vi "MainUI 17.vi"() -> ()   [LabVIEW 2013]
uses:
  eng/trunk/ni/cRIO Master Files/Controls/StateMachineTypeDef.ctl
  eng/trunk/ni/cRIO Master Files/Controls/Up.ctl
  eng/trunk/ni/cRIO Master Files/Controls/Down.ctl
  eng/trunk/ni/cRIO Master Files/Controls/LogState.ctl
  <userlib>/ELL/EventLog/EventLog.lvclass
  <vilib>/Analysis/NI_AALBase.lvlib
  <vilib>/Analysis/3filter.llb/Filter Passband Type.ctl
  <userlib>/ELL/EventLog/Initialize_CSV.vi
  <vilib>/Analysis/3filter.llb/Butterworth Filter (DBL).vi
  eng/trunk/ni/cRIO Master Files/Controls/UserInterfacePages.ctl
  eng/trunk/ni/cRIO Master Files/Controls/SystemControl.ctl
  eng/trunk/ni/cRIO Master Files/Controls/EnergyStorageSelector.ctl
  eng/trunk/ni/cRIO Master Files/Controls/PowerConversionData.ctl
  eng/trunk/ni/cRIO Master Files/Controls/EnergyStorageStringDataArray.ctl
  eng/trunk/ni/cRIO Master Files/Controls/EnergyStorageStringData.ctl
  eng/trunk/ni/cRIO Master Files/Controls/EnergyStorageSystemData.ctl
  eng/trunk/ni/cRIO Master Files/Controls/GensetData.ctl
  Controls/FPGAData.ctl
  eng/trunk/ni/cRIO Master Files/Controls/ModbusInputRegisters.ctl
  eng/trunk/ni/cRIO Master Files/Controls/ModbusHoldingRegisters.ctl
  eng/trunk/ni/cRIO Master Files/Controls/NamedError.ctl
  eng/trunk/ni/cRIO Master Files/Controls/Dial17.ctl
panel:
  in  "Min Cell V":dbl=350.0 min=0.0 max=550.0 format="%#_g V"
  in  "Max Cell V":dbl=672.0 min=3.0 max=750.0 format="%#_g V"
  in  "PS gain P":dbl=0.03
  in  "VI gain P":dbl=55.0
  in  "PS gain I":dbl=0.01
  in  "Cell Limit High":dbl=650.0 min=3.0 max=750.0 format="%#_g V"
  in  "Cell Limit Low":dbl=400.0 min=0.0 max=550.0 format="%#_g V"
  in  "CC gain P":dbl=3.0
  in  "CC gain I":dbl
  in  "HV Setpt":dbl=700.0 format="%#_g V"
  in  "VI gain I":dbl
  in  "Charge Control 2":dbl min=0.0 max=750.0 format="%#_g V"
  in  "Peak Shave 2":dbl min=0.0 max=100.0 format="%#_g kW"
  in  "Up ten PS":T1
  in  "Down ten PS":T2
  in  "Down one PS":T2
  in  "Up one PS":T1
  in  "Up ten MC":T1
  in  "Down ten MC":T2
  in  "Up one MC":T1
  in  "Down one MC":T2
  in  "Manual Current 2":dbl min=-180.0 max=180.0 format="%#_g A"
  in  "Up ten CC":T1
  in  "Down ten CC":T2
  in  "Down one CC":T2
  in  "Up one CC":T1
  out "Samsung":T3
  out "Comap":T3
  out "Interface Data":T3
  out "Log Rate Data":T3
  out "Network Stream":T3
  out "Consumer":T3
  out "Producer":T3
  out "Flush Events":T3
  out "Queue Data Log":T3
  out "Data Logger":T3
  out "DC Voltage":sgl format="%4.1f V"
  out "Samsung Alarm":T4
  out "ComAp Alarm":T4
  out "Siemens Alarm":T4
  in  "Charge Control":bool
  in  "Peak Shave":bool
  out "Exit Program":bool
  in  "Virtual Inertia":bool
  in  "Manual Current":bool
  in  "Stop System":bool
  in  "Start System":bool
  out "Log State":T5
  out "gen eng":u16
  out "gen breaker":u16
  in  "Alarms":bool
  out "Connection Status":bool
  out "Main":bool=TRUE
  in  "Exit Button":bool
  out "Set Points":bool
  out "Metering":bool
  out "Energy Storage":bool
  out "Histogram":bool
  in  "Tab Control":T6=enum."Main"
  out "AC Current 2":sgl(knob) scale=-200.0..200.0 scale format="%3.0fA"
  out "DC Voltage 2":sgl(knob) scale=0.0..750.0 scale format="%3.0fV"
  out "Frequency 2":sgl(knob) scale=45.0..75.0 scale format="%3.0fHz"
  out "DC Current 2":sgl(knob) scale=-200.0..200.0 scale format="%3.0fA"
  out "DC Voltage 3":sgl(knob)=126.0 scale=0.0..750.0 scale format="%3.0fV"
  out "State of Charge":T7=18.015554 scale=0.0..100.0 scale format="%3.0f%"
  out "AC Current":sgl(graph)
  out "Generator Power":sgl(graph)
  out "Generator Frequency":sgl(graph)
  out "Modbus Input Registers":T8 {"Generator Fault Code (30204)" format="%016b"; "Generator Alarm Code (30104)" format="%016b"; "Solar Inverter Fault Code (30203)" format="%016b"; "System Control Fault Code (30202)" format="%016b"; "Power Converter Fault Code (30201)" format="%0d"; "Energy Storage Fault Code (30200)" format="%016b"; "Solar Inverter Alarm Code (30103)" format="%016b"; "System Control Alarm Code (30102)" format="%016b"; "Power Converter Alarm Code (30101)" format="%0d"; "Energy Storage Alarm Code (30100)" format="%016b"; "Fault Word (30053)" format="%016b"; "Alarm Word (30052)" format="%016b"; "Status Word (30051)" format="%016b"}
  out "Modbus Holding Registers":T9={"System Available Capacity (40000)"=600, "System Reserve Percentage (40001)"=200, "System Active Load (40002)"=0, "System Reactive Load (40003)"=0, "Manual Power (40004)"=0, "Manual Current (40005)"=0, "System Watchdog (40006)"=0, "Control Word (40051)"=128, "Clear Faults (40052)"=0} {"Clear Faults (40052)" format="%016b"; "Control Word (40051)" format="%016b"}
  out "Real Time State":string
  out "Drive State":string
  out "E-Stop 2":i32
  out "switch_vert":bool
  out "Power":sgl format="%6.1f kW"
  out "AC Voltage":sgl format="%4.1f V"
  out "icon_batt":bool
  out "switch_batt":bool
  out "switch_gen":bool
  out "switch_drive":bool
  out "switch_load":bool
  out "icon_genset":bool
  out "icon_drive":bool
  out "icon_load":bool
  out "Charge":sgl format="%6.1f %"
  out "DC Current":sgl format="%4.1f A"
  out "DC Voltage":sgl format="%4.1f V"
  out "DC Voltage":sgl format="%4.1f V"
  out "AC Current":sgl format="%4.1f A"
  out "Battery":sgl format="%4.1f V"
  out "Power":dbl format="%6.1f kW"
  out "Frequency":sgl format="%6.1f Hz"
  out "Load":sgl format="%6.1f %"
  out "Temperature":sgl format="%6.1f C"
  out "Power":dbl format="%6.1f kW"
  in  "Clear Alarms":bool
  in  "Stop Log":bool
  out "Alarm Display":string[](array[string])
  out "Alarm Loop":bool
  out "E-Stop":bool
  out "ES System Data":T10
  out "ES String Data":T11
  out "PC Data":T13
  out "FPGA Data":T14
  # "Control Panel"
  # "10"
  # "1"
  # "10"
  # "1"
  # "10"
  # "1"
  # "Charge Limits"
  # "PID Controls"
  # "Energy Storage"
  # "Power Conversion"
  # "System BMS Status"
  # "Rack 1 Status"
  # "Rack 2 Status"
  # "Ioxus UltraCapacitors"
  # "Generator"
  # "Site Load"
  # "Energy Storage"
  # "Power Conversion"
  # "Toshiba"
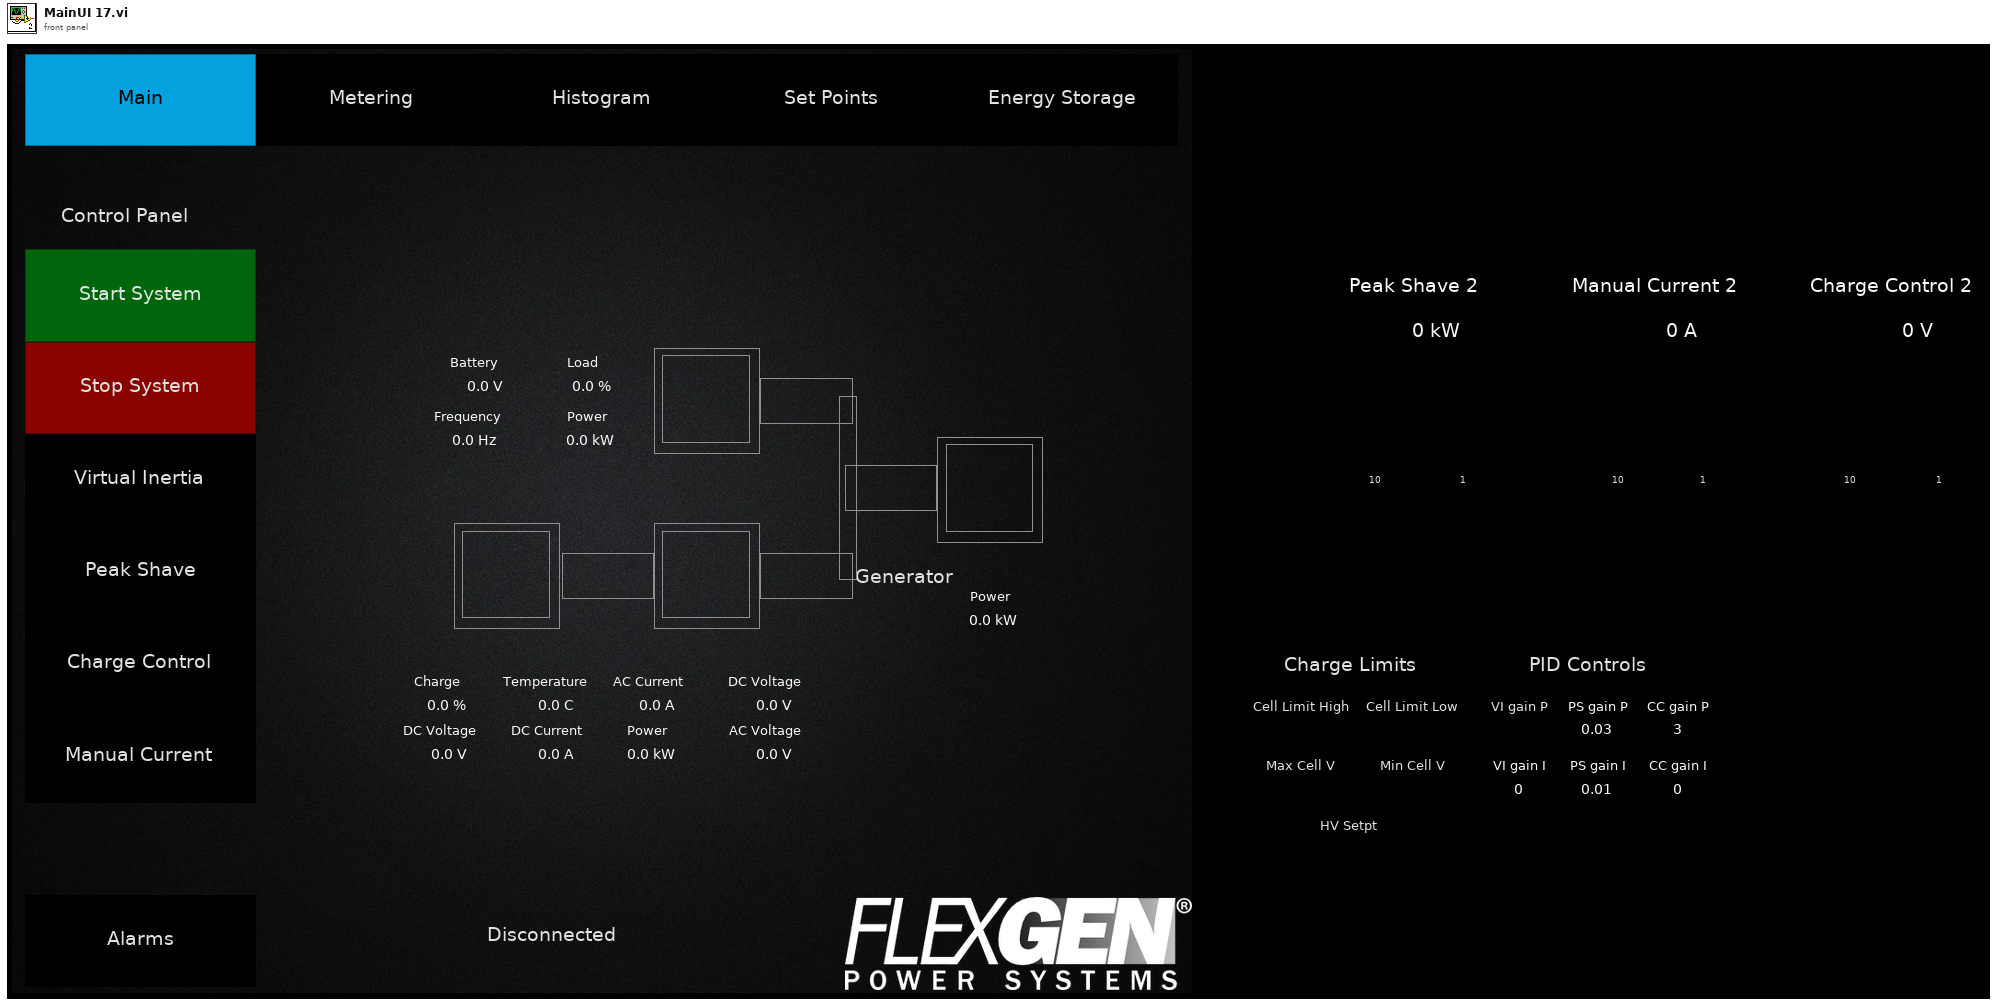
[diagram p1: front panel]
types:
  T1 = typedef "Up.ctl" = bool
  T2 = typedef "Down.ctl" = bool
  T3 = typedef "NamedError.ctl" = cluster{"status":bool, "code":i32, "source":string, "Name":string}
  T4 = cluster{"Fault?":bool, "Alarm?":bool, "Message":string}
  T5 = typedef "LogState.ctl" = enum16{"Rotate Log", "Log Data", "Wait", "Close File", "Generate Filename", "Create New File"}
  T6 = typedef "UserInterfacePages.ctl" = enum32{"Metering", "Histogram", "Set Points", "Samsung", "Ioxus", "Main", "Alarms", "Toshiba", "Siemens"}
  T7 = typedef "Dial17.ctl" = sgl
  T8 = typedef "ModbusInputRegisters.ctl" = cluster{"Energy Remaining (30000)":u16, "Charging Time Remaining (30001)":u16, "Discharging Time Remaining (30002)":u16, "Energy Storage Voltage (30003)":u16, "Energy Storage Current (30004)":i16, "SSG Frequency (30005)":u16, "SSG Total Voltage (30006)":u16, "SSG Total Active Power (30007)":i16, "SSG Total Apparent Power (30008)":i16, "SSG Active Power (L1) (30009)":i16, "SSG Active Power (L2) (30010)":i16, "SSG Active Power (L3) (30011)":i16, "SSG Apparent Power (L1) (30012)":i16, "SSG Apparent Power (L2) (30013)":i16, "SSG Apparent Power (L3) (30014)":i16, "SSG Output Voltage (L1-L2) (30015)":u16, "SSG Output Voltage (L2-L3) (30016)":u16, "SSG Output Voltage (L3-L1) (30017)":u16, "SSG Output Voltage (L1) (30018)":u16, "SSG Output Voltage (L2) (30019)":u16, "SSG Output Voltage (L3) (30020)":u16, "SSG Output Current (L1) (30021)":i16, "SSG Output Current  (L2) (30022)":i16, "SSG Output Current (L3) (30023)":i16, "Energy Storage Temperature (30024)":i16, "Power Converter Temperature (30025)":i16, "Solar Inverter Power (30026)":u16, "Gen Frequency (30027)":u16, "Gen Total Voltage (30028)":u16, "Gen Total Active Power (30029)":i16, "Gen Total Apparent Power (30030)":i16, "Gen Active Power (L1) (30031)":i16, "Gen Active Power (L2) (30032)":i16, "Gen Active Power (L3) (30033)":i16, "Gen Apparent Power (L1) (30034)":i16, "Gen Apparent Power (L2) (30035)":i16, "Gen Apparent Power (L3) (30036)":i16, "Gen Output Voltage (L1-L2) (30037)":u16, "Gen Output Voltage (L2-L3) (30038)":u16, "Gen Output Voltage (L3-L1) (30039)":u16, "Gen Output Voltage (L1) (30040)":u16, "Gen Output Voltage (L2) (30041)":u16, "Gen Output Voltage (L3) (30042)":u16, "Gen Output Current (L1) (30043)":i16, "Gen Output Current  (L2) (30044)":i16, "Gen Output Current (L3) (30045)":i16, "Software Revision (30050)":u16, "Status Word (30051)":u16, "Alarm Word (30052)":u16, "Fault Word (30053)":u16, "Energy Storage Alarm Code (30100)":u16, "Power Converter Alarm Code (30101)":u16, "System Control Alarm Code (30102)":u16, "Solar Inverter Alarm Code (30103)":u16, "Energy Storage Fault Code (30200)":u16, "Power Converter Fault Code (30201)":u16, "System Control Fault Code (30202)":u16, "Solar Inverter Fault Code (30203)":u16, "Generator Alarm Code (30104)":u16, "Generator Fault Code (30204)":u16}
  T9 = typedef "ModbusHoldingRegisters.ctl" = cluster{"System Available Capacity (40000)":u16, "System Reserve Percentage (40001)":u16, "System Active Load (40002)":i16, "System Reactive Load (40003)":i16, "Manual Power (40004)":i16, "Manual Current (40005)":i16, "System Watchdog (40006)":u16, "Control Word (40051)":u16, "Clear Faults (40052)":u16}
  T10 = typedef "EnergyStorageSystemData.ctl" = cluster{"Voltage":sgl, "Current":sgl, "SOC Avg":sgl, "Faults":u16, "Alarms":u16, "Number of Strings":u16, "Max Temp":i16, "Min Temp":i16, "Max Cell Voltage":sgl, "Min Cell Voltage":sgl, "Energy Capacity (kWh)":sgl, "Energy Remaining (kWh)":sgl, "String Code":u16, "SOC Min":sgl, "SOC Max":sgl}
  T11 = typedef "EnergyStorageStringDataArray.ctl" = T12[]
  T12 = typedef "EnergyStorageStringData.ctl" = cluster{"Voltage":sgl, "State of Charge":sgl, "Current":sgl, "Temperature Min":i16, "Temperature Max":i16, "Faults":u16, "Alarms":u16, "String Number":u16, "Contactor Status":bool, "String Ready?":bool, "Cells Balancing":bool, "Cell V Max":dbl, "Cell V Min":dbl}
  T13 = typedef "PowerConversionData.ctl" = cluster{"Active Power":sgl, "Reactive Power":sgl, "AC Current":sgl, "DC Current":sgl, "AC Voltage":sgl, "DC Voltage":sgl, "Temperature":sgl, "Alarms":u16, "Faults":u16, "Status":u16}
  T14 = typedef "FPGAData.ctl" = cluster{"SSG Frequency":sgl, "SSG Total Voltage":dbl, "SSG Active Power":sgl, "SSG Apparent Power":sgl, "SSG Active Power (L1)":dbl, "SSG Active Power (L2)":dbl, "SSG Active Power (L3)":dbl, "SSG Apparent Power (L1)":dbl, "SSG Apparent Power (L2)":dbl, "SSG Apparent Power (L3)":dbl, "SSG Vrms (L1-L2)":dbl, "SSG Vrms (L2-L3)":dbl, "SSG Vrms (L3-L1)":dbl, "SSG Vrms (L1)":dbl, "SSG Vrms (L2)":dbl, "SSG Vrms (L3)":dbl, "SSG Arms (L1)":dbl, "SSG Arms (L2)":dbl, "SSG Arms (L3)":dbl, "Gen Frequency":sgl, "Gen Total Voltage":dbl, "Gen Active Power":sgl, "Gen Apparent Power":sgl, "Gen Active Power (L1)":dbl, "Gen Active Power (L2)":dbl, "Gen Active Power (L3)":dbl, "Gen Apparent Power (L1)":dbl, "Gen Apparent Power (L2)":dbl, "Gen Apparent Power (L3)":dbl, "Gen Vrms (L1-L2)":dbl, "Gen Vrms (L2-L3)":dbl, "Gen Vrms (L3-L1)":dbl, "Gen Vrms (L1)":dbl, "Gen Vrms (L2)":dbl, "Gen Vrms (L3)":dbl, "Gen Arms (L1)":dbl, "Gen Arms (L2)":dbl, "Gen Arms (L3)":dbl, "ES Vdc 1":sgl, "ES Vdc 2":sgl, "Load %":sgl, "Load Imbalance %":sgl, "E-Stop":bool, "Battle Short":bool, "Auto Start":bool, "Gen Contactor":bool, "ES Relay 1":bool, "ES Relay 2":bool, "NFT-N Contactor":bool, "NFT-G Contactor ":bool, "ES Relay 3":bool, "ES Relay 4":bool, "ES Relay 5":bool, "ES Relay 6":bool, "ES Vdc 3":sgl, "ES Vdc 4":sgl, "ES Vdc 5":sgl, "ES Vdc 6":sgl}
  T15 = typedef "StateMachineTypeDef.ctl" = enum16{"Idle", "Initialize", "Alarm Clicked", "go to Set Points", "go to Energy Storage", "go to Power Conversion ", "go to Histogram", "go to Main", "go to Metering", "Enable Charge Control", "Enable External Control", "Enable Manual Current", "Enable Peak Shave", "Disable Virtual Inertia", "Start System", "Stop System", "Shutdown", "Error"}
  T16 = typedef "EnergyStorageSelector.ctl" = enum16{"Other", "Toshiba", "Ioxus", "Samsung"}
  T17 = typedef "NI_AALBase.lvlib/Filter Passband Type.ctl" = enum32{"Lowpass", "Highpass", "Bandpass", "Bandstop"}
  T18 = typedef "FPGAData.ctl" = cluster{"SSG Frequency":sgl, "SSG Total Voltage":dbl, "SSG Active Power":sgl, "SSG Apparent Power":sgl, "SSG Active Power (L1)":dbl, "SSG Active Power (L2)":dbl, "SSG Active Power (L3)":dbl, "SSG Apparent Power (L1)":dbl, "SSG Apparent Power (L2)":dbl, "SSG Apparent Power (L3)":dbl, "SSG Vrms (L1-L2)":dbl, "SSG Vrms (L2-L3)":dbl, "SSG Vrms (L3-L1)":dbl, "SSG Vrms (L1)":dbl, "SSG Vrms (L2)":dbl, "SSG Vrms (L3)":dbl, "SSG Arms (L1)":dbl, "SSG Arms (L2)":dbl, "SSG Arms (L3)":dbl, "Gen Frequency":sgl, "Gen Total Voltage":dbl, "Gen Active Power":sgl, "Gen Apparent Power":sgl, "Gen Active Power (L1)":dbl, "Gen Active Power (L2)":dbl, "Gen Active Power (L3)":dbl, "Gen Apparent Power (L1)":dbl, "Gen Apparent Power (L2)":dbl, "Gen Apparent Power (L3)":dbl, "Gen Vrms (L1-L2)":dbl, "Gen Vrms (L2-L3)":dbl, "Gen Vrms (L3-L1)":dbl, "Gen Vrms (L1)":dbl, "Gen Vrms (L2)":dbl, "Gen Vrms (L3)":dbl, "Gen Arms (L1)":dbl, "Gen Arms (L2)":dbl, "Gen Arms (L3)":dbl, "ES Vdc String 1":sgl, "ES Vdc String 2":sgl, "Load %":sgl, "Load Imbalance %":sgl, "E-Stop":bool, "Battle Short":bool, "Auto Start":bool, "Gen Contactor":bool, "Battery Relay 1":bool, "Battery Relay 2":bool, "NFT-N Contactor":bool, "NFT-G Contactor ":bool}
  T19 = typedef "GensetData.ctl" = cluster{"Alarm Array":u16[], "Power":i16, "Frequency":u16, "Battery":i16, "Engine State":u16, "Breaker State":u16, "Load %":i16}
  T20 = cluster{"status":bool, "code":i32, "source":string, "Name":string}[]
  T21 = cluster{"Fault?":bool, "Alarm?":bool, "Message":string}[]
  T22 = typedef "SystemControl.ctl" = cluster{"Start":bool, "Stop":bool, "Power System Enable":bool, "SSG Control":bool, "Virtual Inertia":bool, "Manual Current":bool, "Peak Shave":bool, "Spot Generation":bool, "Charge Control":bool, "Watchdog":bool, "ComAp Fault":bool, "Clear Gen Faults":bool, "Clear PV Faults":bool, "Clear System Faults":bool, "Clear PC Faults":bool, "Clear ES Faults":bool, "Clear Watchdog Faults":bool, "Peak Shave Value":dbl, "Manual Current Value":dbl, "Charge Control Value":dbl, "Gen Capacity":dbl, "Gen Reserve":dbl, "VI gain P":dbl, "CC gain P":dbl, "CC gain I":dbl}
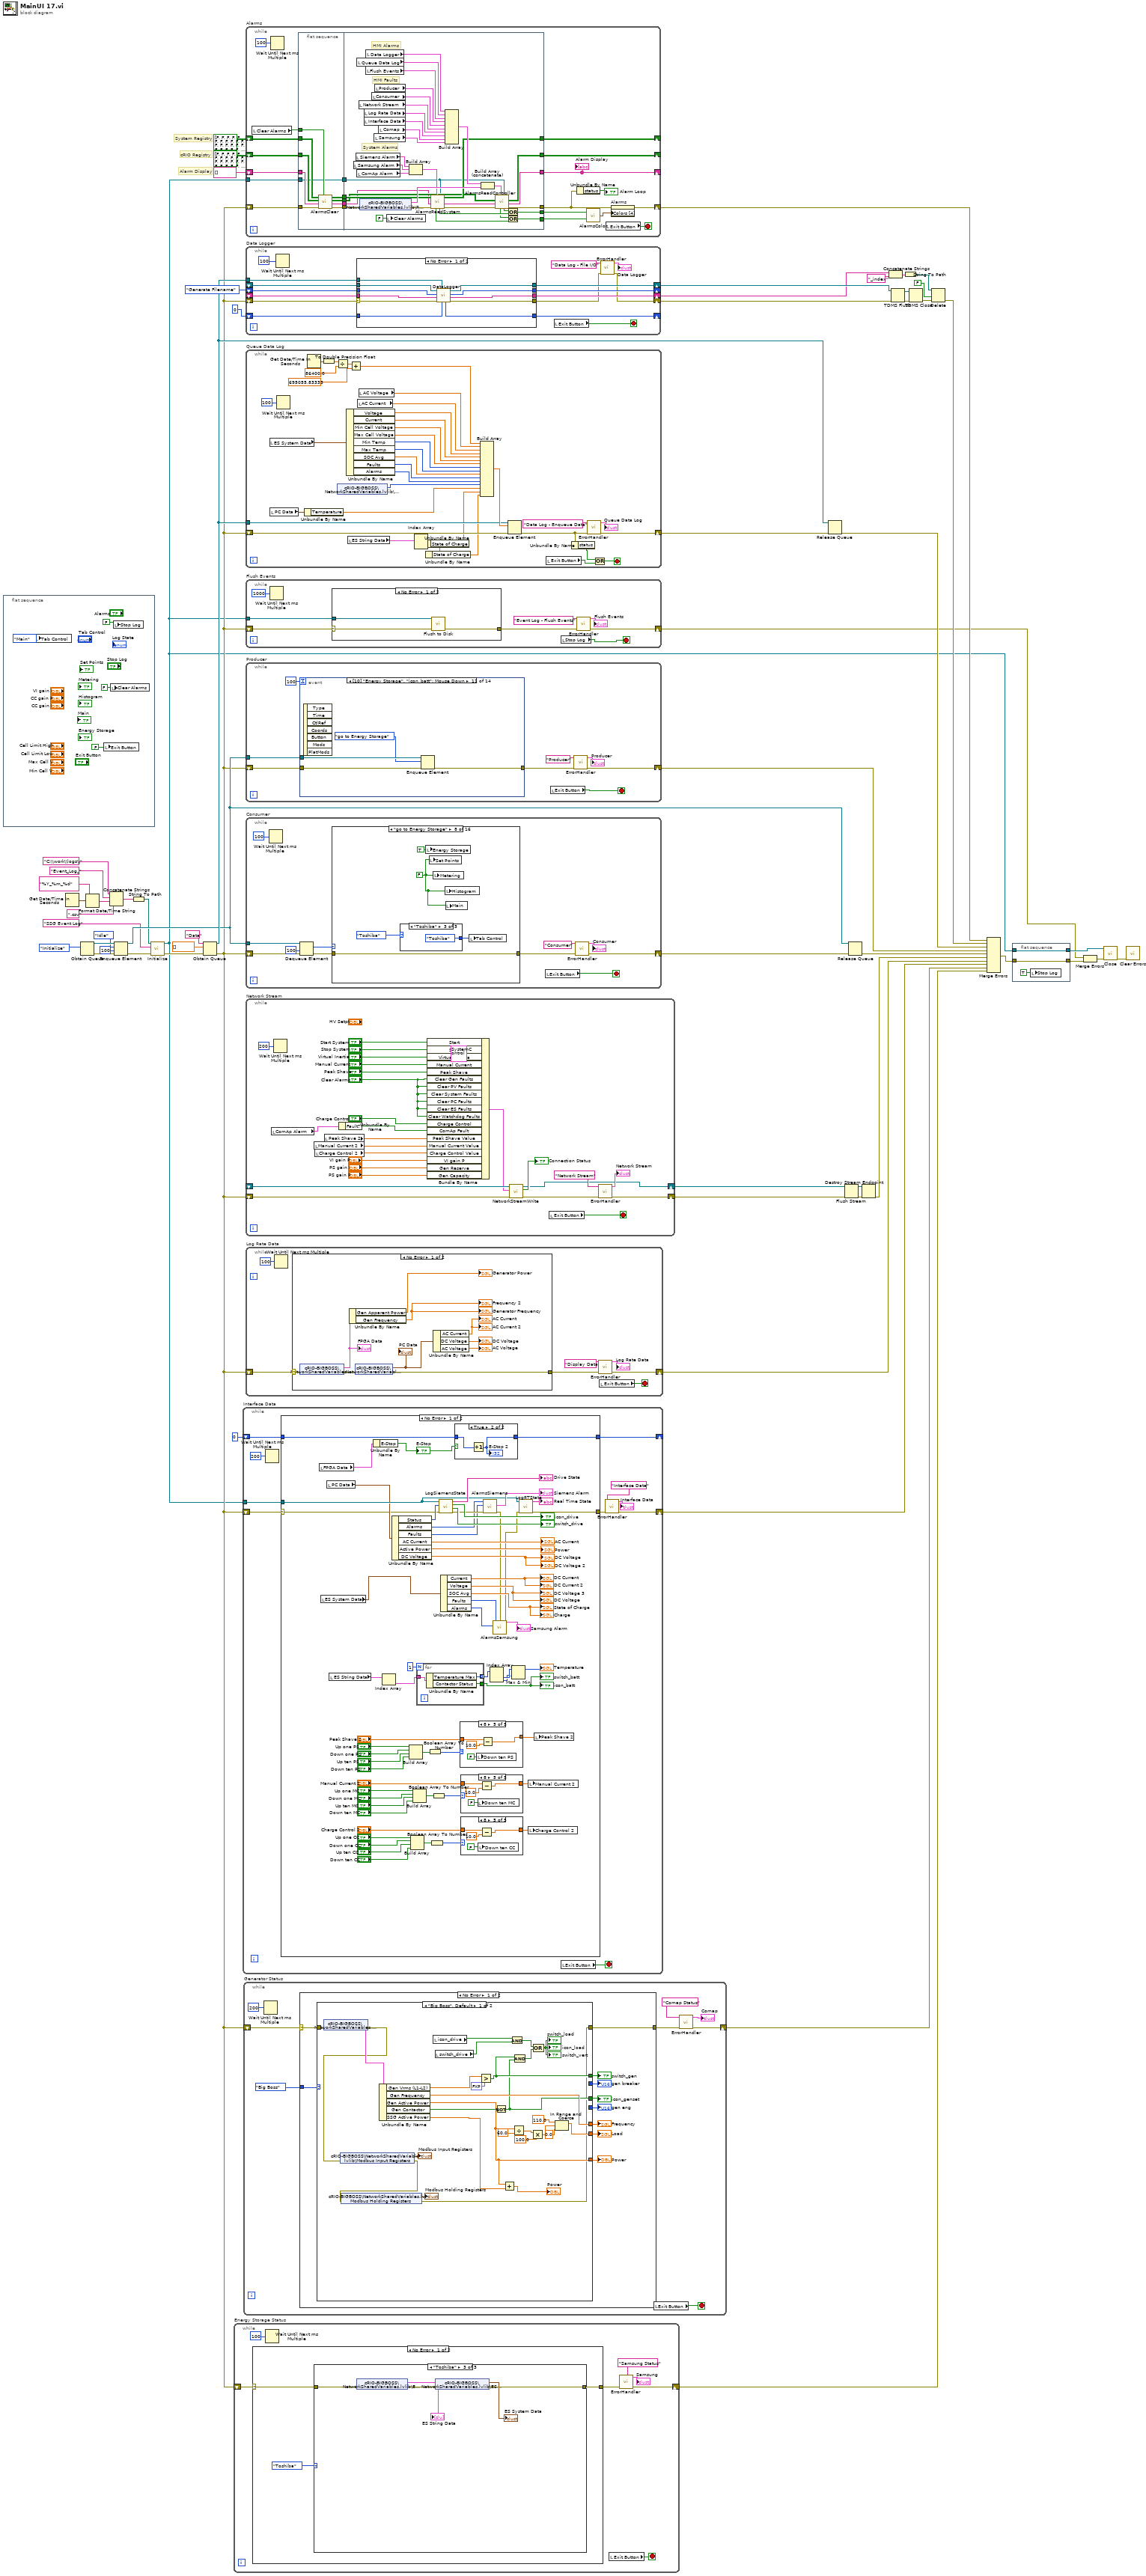
[diagram p0: block diagram]
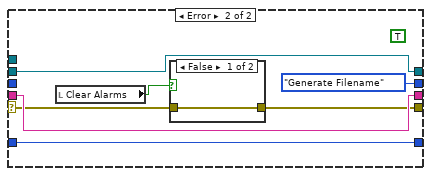
[diagram p2: hidden frame]
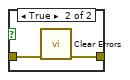
[diagram p3: hidden frame]
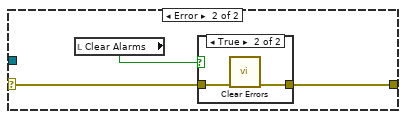
[diagram p4: hidden frame]
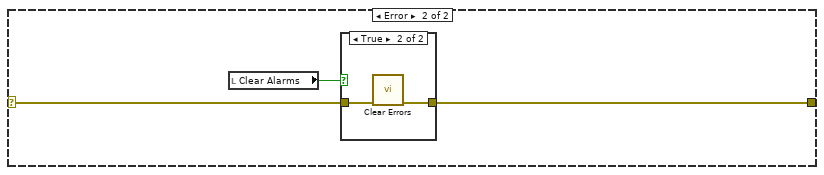
[diagram p8: hidden frame]
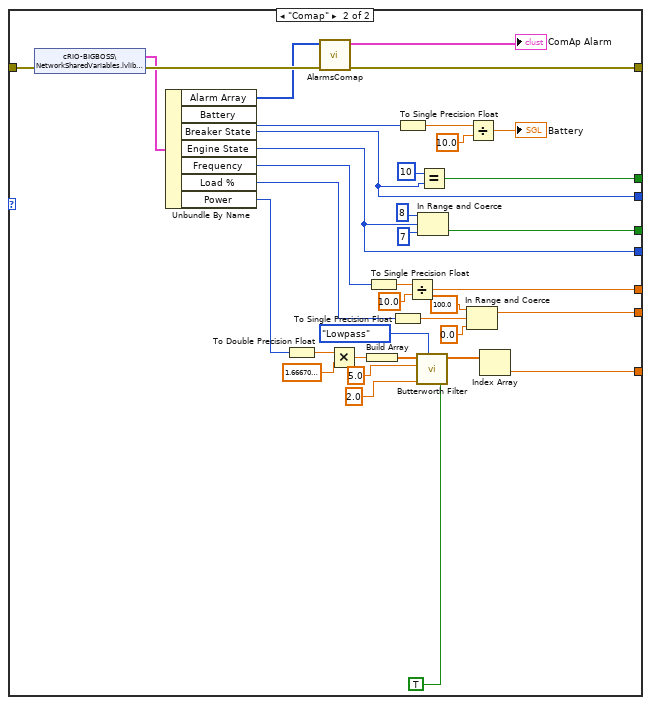
[diagram p10: hidden frame]
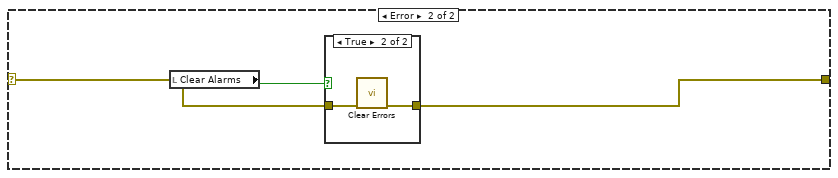
[diagram p11: hidden frame]
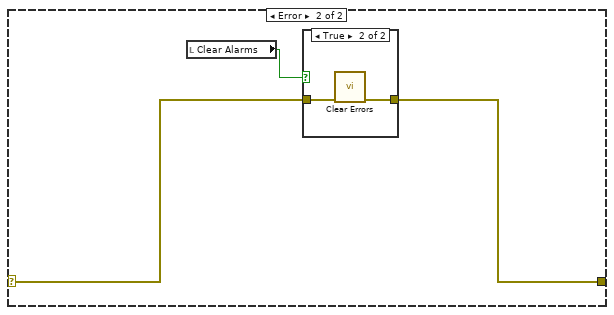
[diagram p13: hidden frame]
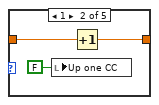
[diagram p16: hidden frame]
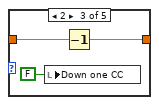
[diagram p17: hidden frame]
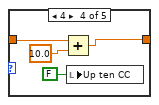
[diagram p18: hidden frame]
diagram:
  # "Alarm Display"
  # "System Registry"
  # "cRIO Registry"
  n1 = flat-sequence {
    frame #0 {
      n2 = local write "Tab Control"(UserInterfacePages."Main" ("Tab Control")) -> ()
      n3 = local write "Exit Button"(FALSE ("Stop Button")) -> ()
      n4 = local write "Clear Alarms"(FALSE ("Clear Errors")) -> ()
      n5 = local write "Stop Log"(FALSE ("Stop Log")) -> ()
    }
  }
  n6 = Get Date/Time In Seconds() -> (seconds since 1Jan1904=w38:timestamp)
  n7 = Obtain Queue(element data type=StateMachineTypeDef."Initialize") -> (queue out=w58:refnum<queue>, error out=w59:errorcluster)  [unwired: 4 in, 1 out]
  n8 = Format Date/Time String(time format string (%c)="%Y_%m_%d", seconds (now)=w38) -> (date/time string=w37:string)  [unwired: 1 in]
  n9 = Concatenate Strings("C:\\work\\logs\\" ("string"), "Event_Log_" ("string"), w37, ".csv" ("string")) -> (w35:string)
  n10 = Enqueue Element(queue=w58, element=StateMachineTypeDef."Idle", timeout in ms (-1)=100, error in (no error)=w59) -> (queue out=w36:refnum<queue>, error out=w27:errorcluster)  [unwired: 1 out]
  n11 = String To Path(string=w35) -> (path=w34:path)
  n12 = call-poly <userlib>:"Initialize.vi"("error in (no error)"=w27, "Description"="SSG Event Log", "Path"=w34) -> ("error out"=w26:errorcluster, "EventLog ref"=w1:refnum<class "EventLog.lvclass">)  [unwired: 7 in]
  n13 = Obtain Queue(name (unnamed)="Data", element data type=dbl[] [] ("appended array"), error in (no error)=w26) -> (queue out=w48:refnum<queue>, error out=w13:errorcluster)  [unwired: 2 in, 1 out]
  n14 = while "Energy Storage Status" {
    shift-right: [w65] -> w19
    shift-left: w13 -> [w69]
    stop <- w70 stop-if-true
    n15 = case shown="No Error" w69 {
      selector: w69 -> [w73 w83]
      tunnel: [w74 w82] -> w68
      frame No Error {
        n16 = case shown="\"Toshiba\"" EnergyStorageSelector."Toshiba" ("Energy Storage Selector") {
          tunnel: w73 -> [w75 w76 w79]
          tunnel: [w75 w76 w81] -> w74
          frame "Other", Default {
          }
          frame "Samsung" {
          }
          frame "Toshiba" {
            n17 = shared-variable "cRIO-BIGBOSS\\NetworkSharedVariables.lvlib\\ES String Data"(error in=w79) -> (→"ES String Data":T11, error out=w78:errorcluster)
            n18 = shared-variable "cRIO-BIGBOSS\\NetworkSharedVariables.lvlib\\ES System Data"(error in=w78) -> (→"ES System Data":T10, error out=w81:errorcluster)
          }
        }
      }
      frame Error {
        n19 = local read "Clear Alarms"() -> (w84:bool)
        n20 = case shown="True" w84 {
          tunnel: w83 -> [w85 w87]
          tunnel: [w85 w86] -> w82
          frame False {
          }
          frame True {
            n21 = call <vilib>:"Clear Errors.vi"("error in (no error)"=w87) -> ("error out"=w86:errorcluster)  [unwired: 6 in]
          }
        }
      }
    }
    n22 = Wait Until Next ms Multiple(millisecond multiple=u32 100 ("milliseconds to wait")) -> ()  [unwired: 1 out]
    n23 = local read "Exit Button"() -> (w70:bool)
    n24 = call "ErrorHandler.vi"("Error In"=w68, "Name"="Samsung Status") -> ("Error Out"=w65:errorcluster, "Named Error Out"=→"Samsung":T3)  [unwired: 6 in]
  }
  n25 = while "Interface Data" {
    shift-right: [w88] -> w14
    shift-left: w13 -> [w94]
    tunnel: w1 -> [w96]
    shift-right: [w92] -> _
    shift-left: 0 -> [w93]
    stop <- w95 stop-if-true
    n26 = Wait Until Next ms Multiple(millisecond multiple=u32 200 ("milliseconds to wait")) -> ()  [unwired: 1 out]
    n27 = case shown="No Error" w94 {
      selector: w94 -> [w98 w211]
      tunnel: w96 -> [w126 _]
      tunnel: [w132 w210] -> w90
      tunnel: w93 -> [w142 w213]
      tunnel: [w141 w213] -> w92
      frame No Error {
        n28 = local read "FPGA Data"() -> (w99:T14)
        n29 = local read "ES System Data"() -> (w104:T10)
        n30 = local read "PC Data"() -> (w100:T13)
        n31 = local read "ES String Data"() -> (w103:T11)
        n32 = Unbundle By Name(w99) -> ("E-Stop"=w105:bool)
        "E-Stop" <- w105
        n33 = Index Array(array=w103) -> (element=w102:T12)  [unwired: 1 in]
        n34 = Unbundle By Name(w100) -> ("Status"=w111:u16, "Alarms"=w112:u16, "Faults"=w113:u16, "AC Current"=→"AC Current":sgl, "Active Power"=→"Power":sgl, "DC Voltage"=→"DC Voltage" →"DC Voltage 2":sgl)
        n35 = Build Array("Up one PS", "Down one PS", "Up ten PS", "Down ten PS") -> (w146:T2[])
        n36 = Build Array("Up one CC", "Down one CC", "Up ten CC", "Down ten CC") -> (w136:T2[])
        n37 = Build Array("Up one MC", "Down one MC", "Up ten MC", "Down ten MC") -> (w153:T2[])
        n38 = for {
          N: 1 -> [_]
          tunnel: w102 -> [w161]
          tunnel: [w160] -> w117 mode=indexing
          tunnel: [w159] -> w114
          n39 = Unbundle By Name(w161) -> ("Temperature Max"=w160:i16, "Contactor Status"=w159:bool)
        }
        "switch_batt" <- w114
        "icon_batt" <- w114
        n40 = Boolean Array To Number(Boolean array=w146) -> (number=w145:u32)
        n41 = Boolean Array To Number(Boolean array=w136) -> (number=w135:u32)
        n42 = Boolean Array To Number(Boolean array=w153) -> (number=w154:u32)
        n43 = call "LogSiemensState.vi"("Error In"=w98, "pb Status In"=w111, "EventLog ref"=w126) -> ("Error Out"=w125:errorcluster, "Switch Out"=→"switch_drive":bool, "Icon Out"=→"icon_drive":bool, "State Out"=→"Drive State":string)  [unwired: 1 in]
        n44 = Unbundle By Name(w104) -> ("Current"=→"DC Current" →"DC Current 2":sgl, "Voltage"=→"DC Voltage" →"DC Voltage 3":sgl, "SOC Avg"=→"Charge" →"State of Charge":sgl, "Faults"=w109:u16, "Alarms"=w108:u16)
        n45 = case shown="True" w105 {
          tunnel: w142 -> [w177 w179]
          tunnel: [w177 w178] -> w141
          frame False {
          }
          frame True {
            n46 = Increment(x=w179) -> (x+1=w178:i32)
            "E-Stop 2" <- w178
          }
        }
        n47 = case shown="8" w145 {
          tunnel: [w180 w183 w186 w189 w194] -> w144
          tunnel: "Peak Shave 2" -> [w180 w181 w184 w187 w191]
          frame 0, Default {
          }
          frame 1 {
            n48 = Increment(x=w181) -> (x+1=w183:dbl)
            n49 = local write "Up one PS"(T1 FALSE ("Up one 2")) -> ()
          }
          frame 2 {
            n50 = local write "Down one PS"(T2 FALSE ("Down one 2")) -> ()
            n51 = Decrement(x=w184) -> (x-1=w186:dbl)
          }
          frame 4 {
            n52 = Add(x=w187, y=10.0) -> (x+y=w189:dbl)
            n53 = local write "Up ten PS"(T1 FALSE ("Up ten 2")) -> ()
          }
          frame 8 {
            n54 = local write "Down ten PS"(T2 FALSE ("Down ten 2")) -> ()
            n55 = Subtract(x=w191, y=10.0) -> (x-y=w194:dbl)
          }
        }
        n56 = case shown="8" w154 {
          tunnel: [w195 w196 w200 w202 w207] -> w152
          tunnel: "Manual Current 2" -> [w195 w197 w201 w204 w208]
          frame 0, Default {
          }
          frame 1 {
            n57 = local write "Up one MC"(T1 FALSE ("Up one")) -> ()
            n58 = Increment(x=w197) -> (x+1=w196:dbl)
          }
          frame 2 {
            n59 = local write "Down one MC"(T2 FALSE ("Down one")) -> ()
            n60 = Decrement(x=w201) -> (x-1=w200:dbl)
          }
          frame 4 {
            n61 = local write "Up ten MC"(T1 FALSE ("Up ten")) -> ()
            n62 = Add(x=w204, y=10.0) -> (x+y=w202:dbl)
          }
          frame 8 {
            n63 = local write "Down ten MC"(T2 FALSE ("Down ten")) -> ()
            n64 = Subtract(x=w208, y=10.0) -> (x-y=w207:dbl)
          }
        }
        n65 = case shown="8" w135 {
          tunnel: "Charge Control 2" -> [w162 w165 w168 w172 w176]
          tunnel: [w162 w164 w167 w171 w174] -> w133
          frame 0, Default {
          }
          frame 1 {
            n66 = local write "Up one CC"(T1 FALSE ("Up one CC")) -> ()
            n67 = Increment(x=w165) -> (x+1=w164:dbl)
          }
          frame 2 {
            n68 = local write "Down one CC"(T2 FALSE ("Down one CC")) -> ()
            n69 = Decrement(x=w168) -> (x-1=w167:dbl)
          }
          frame 4 {
            n70 = Add(x=w172, y=10.0) -> (x+y=w171:dbl)
            n71 = local write "Up ten CC"(T1 FALSE ("Up ten CC")) -> ()
          }
          frame 8 {
            n72 = local write "Down ten CC"(T2 FALSE ("Down ten CC")) -> ()
            n73 = Subtract(x=w176, y=10.0) -> (x-y=w174:dbl)
          }
        }
        n74 = call "AlarmsSiemens.vi"("Error In"=w125, "pb Fault Code"=w113, "pb Alarm Code"=w112) -> ("Error Out"=w107:errorcluster, "System Alarm Out"=→"Siemens Alarm":T4)  [unwired: 3 in]
        n75 = Index Array(array=w117) -> (element #1=w116:i16, element #2=w115:i16)  [unwired: 2 in]
        n76 = call "AlarmsSamsung.vi"("Error In"=w107, "Alarm Code"=w108, "Fault Code"=w109) -> ("Error Out"=w106:errorcluster, "System Alarm Out"=→"Samsung Alarm":T4)  [unwired: 5 in]
        n77 = Max & Min(x=w116, y=w115) -> (max(x,y)=→"Temperature":i16)  [unwired: 1 out]
        n78 = call "LogRTState.vi"("Error In"=w106, "EventLog ref"=w126) -> ("Error Out"=w132:errorcluster, "State Out"=→"Real Time State":string)  [unwired: 4 in]
        n79 = local write "Manual Current 2"(w152) -> ()
        n80 = local write "Charge Control 2"(w133) -> ()
        n81 = local write "Peak Shave 2"(w144) -> ()
      }
      frame Error {
        n82 = local read "Clear Alarms"() -> (w212:bool)
        n83 = case shown="False" w212 {
          tunnel: [w214 w216] -> w210
          tunnel: w211 -> [w214 w215]
          frame False {
          }
          frame True {
            n84 = call <vilib>:"Clear Errors.vi"("error in (no error)"=w215) -> ("error out"=w216:errorcluster)  [unwired: 6 in]
          }
        }
      }
    }
    n85 = local read "Exit Button"() -> (w95:bool)
    n86 = call "ErrorHandler.vi"("Error In"=w90, "Name"="Interface Data") -> ("Error Out"=w88:errorcluster, "Named Error Out"=→"Interface Data":T3)  [unwired: 6 in]
  }
  n87 = while "Generator Status" {
    shift-right: [w218] -> w20
    shift-left: w13 -> [w222]
    stop <- w223 stop-if-true
    n88 = Wait Until Next ms Multiple(millisecond multiple=u32 200 ("milliseconds to wait")) -> ()  [unwired: 1 out]
    n89 = case shown="No Error" w222 {
      selector: w222 -> [w229 w302]
      tunnel: [w226 w301] -> w221
      tunnel: enum16{"Big Boss", "Comap"}."Big Boss" -> [w225 _]
      frame No Error {
        n90 = case shown="\"Big Boss\", Default" w225 {
          tunnel: [w256 w299] -> w234
          tunnel: [w252 w294] -> w233
          tunnel: [w246 w288] -> w232
          tunnel: [w245 w286] -> w231
          tunnel: [w248 w278] -> w230
          tunnel: w229 -> [w262 w273]
          tunnel: [_ w268] -> w228
          tunnel: [_ w267] -> w227
          tunnel: [w237 w263] -> w226
          frame "Big Boss", Default {
            n91 = shared-variable "cRIO-BIGBOSS\\NetworkSharedVariables.lvlib\\FPGA Data"(error in=w262) -> (w261:T18, error out=w239:errorcluster)
            n92 = shared-variable "cRIO-BIGBOSS\\NetworkSharedVariables.lvlib\\Modbus Input Registers"(error in=w239) -> (→"Modbus Input Registers":T8, error out=w238:errorcluster)
            n93 = shared-variable "cRIO-BIGBOSS\\NetworkSharedVariables.lvlib\\Modbus Holding Registers"(error in=w238) -> (→"Modbus Holding Registers":T9, error out=w237:errorcluster)
            n94 = Unbundle By Name(w261) -> ("Gen Vrms (L1-L2)"=w251:dbl, "Gen Frequency"=w252:sgl, "Gen Active Power"=w248:sgl, "Gen Contactor"=w260:bool, "SSG Active Power"=w249:sgl)
            n95 = local read "icon_drive"() -> (w241:bool)
            n96 = local read "switch_drive"() -> (w240:bool)
            n97 = Greater?(x=w251, y=fxp<+,24,10> 160.0) -> (0:w246:bool)
            n98 = Not(x=w260) -> (.not. x?=w245:bool)
            n99 = Add(x=w248, y=w249) -> (x+y=→"Power":sgl)
            n100 = Compound Arithmetic op=AND(w241, w240) -> (w242:bool)
            n101 = Divide(x=w248, y=sgl 60.0) -> (x/y=w258:sgl)
            n102 = Compound Arithmetic op=AND(w246, w245) -> (w244:bool)
            n103 = Multiply(x=w258, y=sgl 100.0) -> (x*y=w255:sgl)
            n104 = Compound Arithmetic op=OR(w242, w244) -> (→"switch_vert" →"switch_load":bool)
            n105 = In Range and Coerce(upper limit=sgl 110.0, x=w255, lower limit=sgl 0.0) -> (coerced(x)=w256:sgl)  [unwired: 1 out]
          }
          frame "Comap" {
            n106 = shared-variable "cRIO-BIGBOSS\\NetworkSharedVariables.lvlib\\Comap Data"(error in=w273) -> (w271:T19, error out=w272:errorcluster)
            n107 = Unbundle By Name(w271) -> ("Alarm Array"=w270:u16[], "Battery"=w269:i16, "Breaker State"=w268:u16, "Engine State"=w267:u16, "Frequency"=w266:u16, "Load %"=w265:i16, "Power"=w264:i16)
            n108 = To Double Precision Float(number=w264) -> (double precision float=w295:dbl)
            n109 = call "AlarmsComap.vi"("Error In"=w272, "Alarm Array"=w270) -> ("Error Out"=w263:errorcluster, "System Alarm Out"=→"ComAp Alarm":T4)  [unwired: 6 in]
            n110 = Multiply(x=w295, y=1.666700005531311) -> (x*y=w281:dbl)
            n111 = Build Array(w281) -> (w280:dbl[])
            n112 = To Single Precision Float(number=w266) -> (single precision float=w292:sgl)
            n113 = To Single Precision Float(number=w265) -> (single precision float=w296:sgl)
            n114 = To Single Precision Float(number=w269) -> (single precision float=w290:sgl)
            n115 = Divide(x=w292, y=sgl 10.0) -> (x/y=w294:sgl)
            n116 = call-poly <vilib>:"Butterworth Filter.vi"("init/cont (init:F)"=TRUE, "filter type"=Filter_Passband_Type."Lowpass", "low cutoff freq: fl"=2.0, "sampling freq: fs"=5.0, "X"=w280) -> ("Filtered X"=w279:dbl[])  [unwired: 3 in, 1 out]
            n117 = In Range and Coerce(upper limit=u16 8, x=w267, lower limit=u16 7) -> (In Range?=w286:bool)  [unwired: 1 out]
            n118 = Equal?(x=u16 10, y=w268) -> (x = y?=w288:bool)
            n119 = In Range and Coerce(upper limit=sgl 100.0, x=w296, lower limit=sgl 0.0) -> (coerced(x)=w299:sgl)  [unwired: 1 out]
            n120 = Divide(x=w290, y=sgl 10.0) -> (x/y=→"Battery":sgl)
            n121 = Index Array(array=w279) -> (element=w278:dbl)  [unwired: 1 in]
          }
        }
        "icon_genset" <- w231
        "switch_gen" <- w232
        "gen breaker" <- w228
        "gen eng" <- w227
        "Power" <- w230
        "Frequency" <- w233
        "Load" <- w234
      }
      frame Error {
        n122 = local read "Clear Alarms"() -> (w300:bool)
        n123 = case shown="True" w300 {
          tunnel: w302 -> [w303 w305]
          tunnel: [w303 w304] -> w301
          frame False {
          }
          frame True {
            n124 = call <vilib>:"Clear Errors.vi"("error in (no error)"=w305) -> ("error out"=w304:errorcluster)  [unwired: 6 in]
          }
        }
      }
    }
    n125 = local read "Exit Button"() -> (w223:bool)
    n126 = call "ErrorHandler.vi"("Error In"=w221, "Name"="Comap Status") -> ("Error Out"=w218:errorcluster, "Named Error Out"=→"Comap":T3)  [unwired: 6 in]
  }
  n127 = while "Alarms" {
    shift-right: [w324] -> w10
    shift-left: w13 -> [w319]
    shift-right: [w314] -> _
    shift-left: string[] [] ("Alarms Display Out") -> [w320]
    shift-right: [w315] -> _
    shift-left: bool[][] [[FALSE, FALSE, FALSE, FALSE, FALSE, FALSE, FALSE, FALSE, FALSE, FALSE, FALSE, FALSE, FALSE, FALSE, FALSE, FALSE, FALSE, FALSE, FALSE, FALSE, FALSE], [FALSE, FALSE, FALSE, FALSE, FALSE, FALSE, FALSE, FALSE, FALSE, FALSE, FALSE, FALSE, FALSE, FALSE, FALSE, FALSE, FALSE, FALSE, FALSE, FALSE, FALSE]] ("Alarm Registry Out") -> [w321]
    shift-right: [w316] -> _
    shift-left: bool[][] [[FALSE, FALSE, FALSE, FALSE, FALSE, FALSE, FALSE, FALSE, FALSE, FALSE, FALSE, FALSE, FALSE, FALSE, FALSE, FALSE, FALSE, FALSE, FALSE, FALSE, FALSE], [FALSE, FALSE, FALSE, FALSE, FALSE, FALSE, FALSE, FALSE, FALSE, FALSE, FALSE, FALSE, FALSE, FALSE, FALSE, FALSE, FALSE, FALSE, FALSE, FALSE, FALSE]] ("Alarm Registry Out") -> [w318]
    tunnel: w1 -> [w306]
    stop <- w327 stop-if-true
    n128 = local read "Clear Alarms"() -> (w322:bool)
    n129 = Wait Until Next ms Multiple(millisecond multiple=u32 100 ("milliseconds to wait")) -> ()  [unwired: 1 out]
    n130 = flat-sequence {
      tunnel: w322 -> [w331]
      tunnel: w321 -> [w333]
      tunnel: w320 -> [w334]
      tunnel: w319 -> [w336]
      tunnel: w318 -> [w332]
      tunnel: [w337] -> w317
      tunnel: [w335] -> w310
      tunnel: [w330] -> w309
      tunnel: [w329] -> w308
      tunnel: w306 -> [w328]
      tunnel: [w328] -> w307
      tunnel: [w344] -> w311
      tunnel: [w350] -> w316
      tunnel: [w345] -> w315
      tunnel: [w339] -> w314
      tunnel: [w372] -> w312
      tunnel: [w373] -> w313
      tunnel: w317 -> [w352]
      tunnel: w310 -> [w371]
      tunnel: w309 -> [w342]
      tunnel: w308 -> [w340]
      tunnel: w307 -> [w338]
      frame #0 {
        n131 = call "AlarmsClear.vi"("Clear Alarms? In"=w331, "Error In"=w336, "Alarm Display In"=w334, "cRIO Registry In"=w333, "System Registry In"=w332) -> ("Error Out"=w335:errorcluster, "Alarms Display Out"=w329:string[], "cRIO Registry Out"=w330:bool[][], "System Registry Out"=w337:bool[][])  [unwired: 1 in]
      }
      frame #1 {
        # "HMI Faults"
        # "HMI Alarms"
        # "System Alarms"
        n132 = local read "Samsung Alarm"() -> (w368:T4)
        n133 = local read "Siemens Alarm"() -> (w367:T4)
        n134 = local read "Queue Data Log"() -> (w358:T3)
        n135 = local read "ComAp Alarm"() -> (w369:T4)
        n136 = local read "Network Stream"() -> (w362:T3)
        n137 = shared-variable "cRIO-BIGBOSS\\NetworkSharedVariables.lvlib\\RT Error Array"(error in=w371) -> (w370:T20, error out=w351:errorcluster)
        n138 = local read "Log Rate Data"() -> (w363:T3)
        n139 = local read "Interface Data"() -> (w364:T3)
        n140 = local read "Flush Events"() -> (w359:T3)
        n141 = local read "Data Logger"() -> (w357:T3)
        n142 = local read "Consumer"() -> (w361:T3)
        n143 = local read "Samsung"() -> (w366:T3)
        n144 = local read "Producer"() -> (w360:T3)
        n145 = local read "Comap"() -> (w365:T3)
        n146 = local write "Clear Alarms"(FALSE ("Clear Errors")) -> ()
        n147 = Build Array(w367, w368, w369) -> (w349:T21)
        n148 = call "AlarmsReadSystem.vi"("EventLog ref"=w338, "System Alarms In"=w349, "Error In"=w351, "Alarms Display In"=w340, "System Registry In"=w352) -> ("Error Out"=w343:errorcluster, "Alarms Display Out"=w341:string[], "System Registry Out"=w350:bool[][], "Faults Out"=w354:bool, "Alarms Out"=w353:bool)  [unwired: 2 in]
        n149 = Build Array(w357, w358, w359, w360, w361, w362, w363, w364, w365, w366) -> (w356:T3[])
        n150 = Build Array (concatenate)(w356, w370) -> (w348:T3[])
        n151 = call "AlarmsReadController.vi"("EventLog ref"=w338, "Alarm Array"=w348, "Error In"=w343, "Alarm Display In"=w341, "cRIO Registry In"=w342) -> ("Error Out"=w344:errorcluster, "Alarms Display Out"=w339:string[], "cRIO Registry Out"=w345:bool[][], "Faults Out"=w347:bool, "Alarms Out"=w346:bool)  [unwired: 2 in]
        n152 = Or(x=w347, y=w354) -> (x .or. y?=w373:bool)
        n153 = Or(x=w346, y=w353) -> (x .or. y?=w372:bool)
      }
    }
    n154 = Unbundle By Name(w311) -> ("status"=→"Alarm Loop":bool)
    n155 = call "AlarmsColor.vi"("Alarms"=w312, "Faults"=w313) -> ("Colors [4]"=w325:cluster{u32, u32}[])
    n156 = local read "Exit Button"() -> (w327:bool)
    n157 = property on="Alarms" class="Bool (strict)"(error in=w311, "Colors [4]"=w325) -> (error out=w324:errorcluster)  [unwired: 1 in, 1 out]
    "Alarm Display" <- w314
  }
  n158 = while "Data Logger" {
    shift-right: [w383] -> w51
    shift-left: _ -> [w382]
    shift-right: [w374] -> w7
    shift-left: w13 -> [w381]
    tunnel: w48 -> [w388]
    shift-right: [w384] -> _
    shift-left: LogState."Generate Filename" ("Log State") -> [w385]
    shift-right: [w386] -> w41
    shift-left: _ -> [w387]
    shift-right: [w379] -> _
    shift-left: 0 ("Filename Counter Out") -> [w378]
    stop <- w380 stop-if-true
    n159 = Wait Until Next ms Multiple(millisecond multiple=u32 100 ("milliseconds to wait")) -> ()  [unwired: 1 out]
    n160 = case shown="No Error" w381 {
      selector: w381 -> [w393 w401]
      tunnel: w388 -> [w394 _]
      tunnel: w387 -> [w396 w405]
      tunnel: [w395 w405] -> w386
      tunnel: w385 -> [w398 _]
      tunnel: [w392 w402] -> w377
      tunnel: [w397 LogState."Generate Filename" ("Log State Out")] -> w384
      tunnel: [w399 w406] -> w383
      tunnel: w382 -> [w400 w406]
      tunnel: [w390 w404] -> w379
      tunnel: w378 -> [w391 w404]
      frame No Error {
        n161 = call "DataLogger.vi"("Filename Counter In"=w391, "Queue In"=w394, "Error In"=w393, "String In"=w396, "Log State In"=w398, "TDMS File In"=w400) -> ("Error Out"=w392:errorcluster, "String Out"=w395:string, "Log State Out"=w397:T5, "TDMS File Out"=w399:refnum<k34>, "Filename Counter Out"=w390:i32)
      }
      frame Error {
        (unwired) TRUE ("Log Event? Out")
        n162 = local read "Clear Alarms"() -> (w403:bool)
        n163 = case shown="False" w403 {
          tunnel: w401 -> [w408 w410]
          tunnel: [w408 w409] -> w402
          frame False {
          }
          frame True {
            n164 = call <vilib>:"Clear Errors.vi"("error in (no error)"=w410) -> ("error out"=w409:errorcluster)  [unwired: 6 in]
          }
        }
      }
    }
    n165 = local read "Exit Button"() -> (w380:bool)
    n166 = call "ErrorHandler.vi"("Error In"=w377, "Name"="Data Log - File I/O") -> ("Error Out"=w374:errorcluster, "Named Error Out"=→"Data Logger":T3)  [unwired: 6 in]
  }
  n167 = while "Queue Data Log" {
    tunnel: w48 -> [w445]
    shift-right: [w431] -> w8
    shift-left: w13 -> [w444]
    stop <- w443 stop-if-true
    n168 = local read "ES System Data"() -> (w430:T10)
    n169 = local read "PC Data"() -> (w418:T13)
    n170 = Wait Until Next ms Multiple(millisecond multiple=u32 100 ("milliseconds to wait")) -> ()  [unwired: 1 out]
    n171 = Unbundle By Name(w418) -> ("Temperature"=w417:sgl)
    n172 = Get Date/Time In Seconds() -> (seconds since 1Jan1904=w436:timestamp)
    n173 = To Double Precision Float(number=w436) -> (double precision float=w439:dbl)
    n174 = Divide(x=w439, y=86400.0) -> (x/y=w440:dbl)
    n175 = shared-variable "cRIO-BIGBOSS\\NetworkSharedVariables.lvlib\\Battery Faults"() -> (w416:u32)  [unwired: 1 in, 1 out]
    n176 = Unbundle By Name(w430) -> ("Voltage"=w427:sgl, "Current"=w426:sgl, "Min Cell Voltage"=w425:sgl, "Max Cell Voltage"=w424:sgl, "Min Temp"=w423:i16, "Max Temp"=w422:i16, "SOC Avg"=w421:sgl, "Faults"=w420:u16, "Alarms"=w419:u16)
    n177 = local read "ES String Data"() -> (w415:T11)
    n178 = Add(x=w440, y=695055.83333) -> (x+y=w435:dbl)
    n179 = local read "AC Current"() -> (w428:sgl)
    n180 = local read "AC Voltage"() -> (w429:sgl)
    n181 = Index Array(array=w415) -> (element #1=w414:T12, element #2=w413:T12)  [unwired: 2 in]
    n182 = Unbundle By Name(w414) -> ("State of Charge"=w412:sgl)
    n183 = Unbundle By Name(w413) -> ("State of Charge"=w411:sgl)
    n184 = Build Array(w435, w429, w428, w427, w426, w425, w424, w423, w422, w421, w420, w419, w416, w417, w412, w411) -> (w446:dbl[])
    n185 = Enqueue Element(queue=w445, element=w446, error in (no error)=w444) -> (error out=w434:errorcluster)  [unwired: 1 in, 2 out]
    n186 = local read "Exit Button"() -> (w442:bool)
    n187 = Unbundle By Name(w434) -> ("status"=w441:bool)
    n188 = call "ErrorHandler.vi"("Error In"=w434, "Name"="Data Log - Enqueue Data") -> ("Error Out"=w431:errorcluster, "Named Error Out"=→"Queue Data Log":T3)  [unwired: 6 in]
    n189 = Or(x=w441, y=w442) -> (x .or. y?=w443:bool)
  }
  n190 = while "Flush Events" {
    tunnel: w1 -> [w455]
    shift-right: [w448] -> w9
    shift-left: w13 -> [w453]
    stop <- w452 stop-if-true
    n191 = Wait Until Next ms Multiple(millisecond multiple=u32 1000 ("milliseconds to wait")) -> ()  [unwired: 1 out]
    n192 = case shown="No Error" w453 {
      selector: w453 -> [w456 w461]
      tunnel: [w458 w460] -> w451
      tunnel: w455 -> [w457 _]
      frame No Error {
        n193 = call <userlib>:"Flush to Disk.vi"("error in (no error)"=w456, "EventLog ref"=w457) -> ("error out"=w458:errorcluster)  [unwired: 8 in, 1 out]
      }
      frame Error {
        n194 = local read "Clear Alarms"() -> (w459:bool)
        n195 = case shown="True" w459 {
          tunnel: w461 -> [w462 w464]
          tunnel: [w462 w463] -> w460
          frame False {
          }
          frame True {
            n196 = call <vilib>:"Clear Errors.vi"("error in (no error)"=w464) -> ("error out"=w463:errorcluster)  [unwired: 6 in]
          }
        }
      }
    }
    n197 = local read "Stop Log"() -> (w452:bool)
    n198 = call "ErrorHandler.vi"("Error In"=w451, "Name"="Event Log - Flush Events") -> ("Error Out"=w448:errorcluster, "Named Error Out"=→"Flush Events":T3)  [unwired: 6 in]
  }
  n199 = while "Producer" {
    tunnel: w36 -> [w470]
    shift-right: [w465] -> w16
    shift-left: w13 -> [w471]
    stop <- w469 stop-if-true
    n200 = event shown="[10] \"Energy Storage\", \"icon_batt\": Mouse Down" {
      selector: _ -> [_ _ _ _ _ _ _ _ _ _ _ _ _ _]
      dyn-events: _ -> [_ _ _ _ _ _ _ _ _ _ _ _ _ _]
      timeout: 100 -> [_ _ _ _ _ _ _ _ _ _ _ _ _ _]
      tunnel: w471 -> [w473 w474 w478 w487 w496 w505 w514 w524 w525 w532 w536 w539 w544 w548]
      tunnel: [w473 w474 w477 w486 w495 w504 w513 w523 w528 w531 w535 w537 w543 w547] -> w468
      tunnel: w470 -> [_ _ w476 w485 w494 w503 w512 w522 w527 w530 w534 w540 w542 w546]
      event Timeout {
        n201 = event-data() -> ()  [unwired: 1 in, 2 out]
      }
      event "Exit Button": Value Change; "Exit Program": Mouse Down {
        n202 = event-data() -> ()  [unwired: 1 in, 3 out]
        n203 = local write "Exit Button"(TRUE ("Stop Button")) -> ()
      }
      event "Start System": Value Change {
        n204 = event-data() -> ("NewVal"=w479:bool)  [unwired: 1 in, 4 out]
        n205 = case shown="False" w479 {
          tunnel: w478 -> [w480 w484]
          tunnel: [w480 w483] -> w477
          tunnel: w476 -> [_ w482]
          frame False {
          }
          frame True {
            n206 = Enqueue Element(queue=w482, element=StateMachineTypeDef."Start System", error in (no error)=w484) -> (error out=w483:errorcluster)  [unwired: 1 in, 2 out]
          }
        }
      }
      event "Peak Shave": Value Change {
        n207 = event-data() -> ("NewVal"=w488:bool)  [unwired: 1 in, 4 out]
        n208 = case shown="True" w488 {
          tunnel: w487 -> [w489 w493]
          tunnel: [w489 w492] -> w486
          tunnel: w485 -> [_ w491]
          frame False {
          }
          frame True {
            n209 = Enqueue Element(queue=w491, element=StateMachineTypeDef."Enable Peak Shave", error in (no error)=w493) -> (error out=w492:errorcluster)  [unwired: 1 in, 2 out]
          }
        }
      }
      event "Charge Control": Value Change {
        n210 = event-data() -> ("NewVal"=w497:bool)  [unwired: 1 in, 4 out]
        n211 = case shown="False" w497 {
          tunnel: w496 -> [w498 w502]
          tunnel: [w498 w501] -> w495
          tunnel: w494 -> [_ w500]
          frame False {
          }
          frame True {
            n212 = Enqueue Element(queue=w500, element=StateMachineTypeDef."Enable Charge Control", error in (no error)=w502) -> (error out=w501:errorcluster)  [unwired: 1 in, 2 out]
          }
        }
      }
      event "Manual Current": Value Change {
        n213 = event-data() -> ("NewVal"=w506:bool)  [unwired: 1 in, 4 out]
        n214 = case shown="False" w506 {
          tunnel: w505 -> [w507 w511]
          tunnel: [w507 w510] -> w504
          tunnel: w503 -> [_ w509]
          frame False {
          }
          frame True {
            n215 = Enqueue Element(queue=w509, element=StateMachineTypeDef."Enable Manual Current", error in (no error)=w511) -> (error out=w510:errorcluster)  [unwired: 1 in, 2 out]
          }
        }
      }
      event "Stop System": Value Change {
        n216 = event-data() -> ("NewVal"=w515:bool)  [unwired: 1 in, 4 out]
        n217 = case shown="True" w515 {
          tunnel: w514 -> [w516 w520]
          tunnel: [w516 w519] -> w513
          tunnel: w512 -> [_ w518]
          frame False {
          }
          frame True {
            n218 = Enqueue Element(queue=w518, element=StateMachineTypeDef."Stop System", error in (no error)=w520) -> (error out=w519:errorcluster)  [unwired: 1 in, 2 out]
          }
        }
      }
      event "Alarms": Mouse Down {
        n219 = event-data() -> ()  [unwired: 1 in, 7 out]
        n220 = Enqueue Element(queue=w522, element=StateMachineTypeDef."Alarm Clicked", error in (no error)=w524) -> (error out=w523:errorcluster)  [unwired: 1 in, 2 out]
      }
      event "Metering": Mouse Down {
        n221 = event-data() -> ()  [unwired: 1 in, 7 out]
        n222 = Enqueue Element(queue=w527, element=StateMachineTypeDef."go to Metering", error in (no error)=w525) -> (error out=w528:errorcluster)  [unwired: 1 in, 2 out]
      }
      event "Histogram": Mouse Down {
        n223 = event-data() -> ()  [unwired: 1 in, 7 out]
        n224 = Enqueue Element(queue=w530, element=StateMachineTypeDef."go to Histogram", error in (no error)=w532) -> (error out=w531:errorcluster)  [unwired: 1 in, 2 out]
      }
      event "Energy Storage", "icon_batt": Mouse Down {
        n225 = event-data() -> ()  [unwired: 1 in, 7 out]
        n226 = Enqueue Element(queue=w534, element=StateMachineTypeDef."go to Energy Storage", error in (no error)=w536) -> (error out=w535:errorcluster)  [unwired: 1 in, 2 out]
      }
      event "icon_drive": Mouse Down {
        n227 = event-data() -> ()  [unwired: 1 in, 7 out]
        n228 = Enqueue Element(queue=w540, element=StateMachineTypeDef."go to Power Conversion ", error in (no error)=w539) -> (error out=w537:errorcluster)  [unwired: 1 in, 2 out]
      }
      event "Set Points": Mouse Down {
        n229 = event-data() -> ()  [unwired: 1 in, 7 out]
        n230 = Enqueue Element(queue=w542, element=StateMachineTypeDef."go to Set Points", error in (no error)=w544) -> (error out=w543:errorcluster)  [unwired: 1 in, 2 out]
      }
      event "Main": Mouse Down {
        n231 = event-data() -> ()  [unwired: 1 in, 7 out]
        n232 = Enqueue Element(queue=w546, element=StateMachineTypeDef."go to Main", error in (no error)=w548) -> (error out=w547:errorcluster)  [unwired: 1 in, 2 out]
      }
    }
    n233 = local read "Exit Button"() -> (w469:bool)
    n234 = call "ErrorHandler.vi"("Error In"=w468, "Name"="Producer") -> ("Error Out"=w465:errorcluster, "Named Error Out"=→"Producer":T3)  [unwired: 6 in]
  }
  n235 = while "Consumer" {
    tunnel: w36 -> [w557]
    shift-right: [w549] -> w15
    shift-left: w13 -> [w559]
    stop <- w553 stop-if-true
    n236 = Wait Until Next ms Multiple(millisecond multiple=u32 100 ("milliseconds to wait")) -> ()  [unwired: 1 out]
    n237 = Dequeue Element(queue=w557, timeout in ms (-1)=100, error in (no error)=w559) -> (element=w556:T15, error out=w558:errorcluster)  [unwired: 2 out]
    n238 = case shown="\"go to Energy Storage\"" w556 {
      tunnel: w558 -> [w560 w564 w567 w568 w569 w573 w576 w582 w587 w591 w595 w597 w598 w600 w603 w605]
      tunnel: [w560 w564 w567 w568 w569 w573 w576 w582 w587 w591 w595 w597 w598 w600 w603 w605] -> w552
      frame "Idle" {
      }
      frame "Initialize" {
        w563 = FALSE
        n239 = local write "Main"(TRUE) -> ()
        n240 = local write "Metering"(w563) -> ()
        n241 = local write "Energy Storage"(w563) -> ()
        n242 = local write "Tab Control"(UserInterfacePages."Main" ("Tab Control")) -> ()
        n243 = local write "Histogram"(w563) -> ()
        n244 = local write "Set Points"(w563) -> ()
      }
      frame "Alarm Clicked" {
        w566 = FALSE
        n245 = local write "Metering"(w566) -> ()
        n246 = local write "Histogram"(w566) -> ()
        n247 = local write "Set Points"(w566) -> ()
        n248 = local write "Tab Control"(UserInterfacePages."Alarms" ("Tab Control")) -> ()
        n249 = local write "Main"(w566) -> ()
        n250 = local write "Energy Storage"(w566) -> ()
      }
      frame "Shutdown" {
      }
      frame "Error", Default {
      }
      frame "go to Set Points" {
        w571 = FALSE ("Setup and Control")
        n251 = local write "Tab Control"(UserInterfacePages."Set Points" ("Tab Control")) -> ()
        n252 = local write "Energy Storage"(w571) -> ()
        n253 = local write "Main"(w571) -> ()
        n254 = local write "Metering"(w571) -> ()
        n255 = local write "Set Points"(TRUE ("Setup and Control")) -> ()
        n256 = local write "Histogram"(w571) -> ()
      }
      frame "go to Metering" {
        w575 = FALSE ("Data Logging")
        n257 = local write "Energy Storage"(w575) -> ()
        n258 = local write "Metering"(TRUE ("Metering")) -> ()
        n259 = local write "Main"(w575) -> ()
        n260 = local write "Tab Control"(UserInterfacePages."Metering" ("Tab Control")) -> ()
        n261 = local write "Set Points"(w575) -> ()
        n262 = local write "Histogram"(w575) -> ()
      }
      frame "go to Energy Storage" {
        w581 = FALSE ("Data Logging")
        n263 = case shown="\"Toshiba\"" EnergyStorageSelector."Toshiba" ("Energy Storage Selector") {
          tunnel: [UserInterfacePages."Samsung" ("Tab Control") UserInterfacePages."Samsung" ("Tab Control") UserInterfacePages."Toshiba" ("Tab Control")] -> w578
          frame "Other", Default {
          }
          frame "Samsung" {
          }
          frame "Toshiba" {
          }
        }
        n264 = local write "Energy Storage"(TRUE ("Data Logging")) -> ()
        n265 = local write "Set Points"(w581) -> ()
        n266 = local write "Metering"(w581) -> ()
        n267 = local write "Histogram"(w581) -> ()
        n268 = local write "Main"(w581) -> ()
        n269 = local write "Tab Control"(w578) -> ()
      }
      frame "go to Power Conversion " {
        n270 = local write "Tab Control"(UserInterfacePages."Siemens" ("Tab Control")) -> ()
      }
      frame "go to Histogram" {
        w589 = FALSE ("AC Bus Status and History")
        n271 = local write "Set Points"(w589) -> ()
        n272 = local write "Energy Storage"(w589) -> ()
        n273 = local write "Metering"(w589) -> ()
        n274 = local write "Tab Control"(UserInterfacePages."Histogram" ("Tab Control")) -> ()
        n275 = local write "Main"(w589) -> ()
        n276 = local write "Histogram"(TRUE ("AC Bus Status and History")) -> ()
      }
      frame "go to Main" {
        w593 = FALSE ("AC Bus Status and History")
        n277 = local write "Tab Control"(UserInterfacePages."Main" ("Tab Control")) -> ()
        n278 = local write "Energy Storage"(w593) -> ()
        n279 = local write "Main"(TRUE ("AC Bus Status and History")) -> ()
        n280 = local write "Set Points"(w593) -> ()
        n281 = local write "Histogram"(w593) -> ()
        n282 = local write "Metering"(w593) -> ()
      }
      frame "Enable Peak Shave" {
        w596 = FALSE
        n283 = local write "Charge Control"(w596) -> ()
        n284 = local write "Manual Current"(w596) -> ()
      }
      frame "Enable Manual Current" {
        w599 = FALSE
        n285 = local write "Peak Shave"(w599) -> ()
        n286 = local write "Charge Control"(w599) -> ()
      }
      frame "Enable Charge Control" {
        w601 = FALSE
        n287 = local write "Peak Shave"(w601) -> ()
        n288 = local write "Manual Current"(w601) -> ()
      }
      frame "Start System" {
        w602 = FALSE
        n289 = local write "Virtual Inertia"(w602) -> ()
        n290 = local write "Manual Current"(w602) -> ()
        n291 = local write "Peak Shave"(w602) -> ()
        n292 = local write "Charge Control"(w602) -> ()
      }
      frame "Stop System" {
        w604 = FALSE ("Start System")
        n293 = local write "Start System"(w604) -> ()
        n294 = local write "Virtual Inertia"(w604) -> ()
        n295 = local write "Manual Current"(w604) -> ()
        n296 = local write "Peak Shave"(w604) -> ()
        n297 = local write "Charge Control"(w604) -> ()
      }
    }
    n298 = local read "Exit Button"() -> (w553:bool)
    n299 = call "ErrorHandler.vi"("Error In"=w552, "Name"="Consumer") -> ("Error Out"=w549:errorcluster, "Named Error Out"=→"Consumer":T3)  [unwired: 6 in]
  }
  n300 = while "Network Stream" {
    shift-right: [w607] -> w12
    shift-left: _ -> [w628]
    shift-right: [w610] -> w17
    shift-left: w13 -> [w630]
    stop <- w631 stop-if-true
    n301 = local read "ComAp Alarm"() -> (w625:T4)
    n302 = Wait Until Next ms Multiple(millisecond multiple=u32 200 ("milliseconds to wait")) -> ()  [unwired: 1 out]
    n303 = local read "Manual Current 2"() -> (w615:dbl)
    n304 = local read "Charge Control 2"() -> (w616:dbl)
    n305 = local read "Peak Shave 2"() -> (w614:dbl)
    n306 = Unbundle By Name(w625) -> ("Fault?"=w617:bool)
    n307 = Bundle By Name(cluster=T22 {"Start"=FALSE, "Stop"=FALSE, "Power System Enable"=FALSE, "SSG Control"=FALSE, "Virtual Inertia"=FALSE, "Manual Current"=FALSE, "Peak Shave"=FALSE, "Spot Generation"=FALSE, "Charge Control"=FALSE, "Watchdog"=FALSE, "ComAp Fault"=FALSE, "Clear Gen Faults"=FALSE, "Clear PV Faults"=FALSE, "Clear System Faults"=FALSE, "Clear PC Faults"=FALSE, "Clear ES Faults"=FALSE, "Clear Watchdog Faults"=FALSE, "Peak Shave Value"=0.0, "Manual Current Value"=0.0, "Charge Control Value"=0.0, "Gen Capacity"=0.0, "Gen Reserve"=0.0, "VI gain P"=0.0, "CC gain P"=0.0, "CC gain I"=0.0} ("System Control 2"), "Start"="Start System", "Stop"="Stop System", "Virtual Inertia"="Virtual Inertia", "Manual Current"="Manual Current", "Peak Shave"="Peak Shave", "Clear Gen Faults"="Clear Alarms", "Clear PV Faults"="Clear Alarms", "Clear System Faults"="Clear Alarms", "Clear PC Faults"="Clear Alarms", "Clear ES Faults"="Clear Alarms", "Clear Watchdog Faults"="Clear Alarms", "Charge Control"="Charge Control", "ComAp Fault"=w617, "Peak Shave Value"=w614, "Manual Current Value"=w615, "Charge Control Value"=w616, "VI gain P"="VI gain P", "Gen Reserve"="PS gain I", "Gen Capacity"="PS gain P") -> (w623:T22)
    n308 = call "NetworkStreamWrite.vi"("Error In"=w630, "Data In"=w623, "Network Stream Ref In"=w628) -> ("Error Out"=w627:errorcluster, "Connected"=→"Connection Status":bool, "Network Stream Ref Out"=w607:refnum<k21>)  [unwired: 6 in]
    n309 = local read "Exit Button"() -> (w631:bool)
    n310 = call "ErrorHandler.vi"("Error In"=w627, "Name"="Network Stream") -> ("Error Out"=w610:errorcluster, "Named Error Out"=→"Network Stream":T3)  [unwired: 6 in]
  }
  n311 = while "Log Rate Data" {
    shift-right: [w633] -> w18
    shift-left: w13 -> [w638]
    stop <- w637 stop-if-true
    n312 = Wait Until Next ms Multiple(millisecond multiple=u32 100 ("milliseconds to wait")) -> ()  [unwired: 1 out]
    n313 = case shown="No Error" w638 {
      selector: w638 -> [w645 w651]
      tunnel: [w646 w650] -> w636
      frame No Error {
        n314 = shared-variable "cRIO-BIGBOSS\\NetworkSharedVariables.lvlib\\FPGA Data"(error in=w645) -> (w643:T18, error out=w644:errorcluster)
        "FPGA Data" <- w643
        n315 = Unbundle By Name(w643) -> ("Gen Apparent Power"=→"Generator Power":sgl, "Gen Frequency"=→"Frequency 2" →"Generator Frequency":sgl)
        n316 = shared-variable "cRIO-BIGBOSS\\NetworkSharedVariables.lvlib\\PC Data"(error in=w644) -> (w649:T13, error out=w646:errorcluster)
        "PC Data" <- w649
        n317 = Unbundle By Name(w649) -> ("AC Current"=→"AC Current" →"AC Current 2":sgl, "DC Voltage"=→"DC Voltage":sgl, "AC Voltage"=→"AC Voltage":sgl)
      }
      frame Error {
        n318 = local read "Clear Alarms"() -> (w652:bool)
        n319 = case shown="True" w652 {
          tunnel: w651 -> [w653 w655]
          tunnel: [w653 w654] -> w650
          frame False {
          }
          frame True {
            n320 = call <vilib>:"Clear Errors.vi"("error in (no error)"=w655) -> ("error out"=w654:errorcluster)  [unwired: 6 in]
          }
        }
      }
    }
    n321 = call "ErrorHandler.vi"("Error In"=w636, "Name"="Display Data") -> ("Error Out"=w633:errorcluster, "Named Error Out"=→"Log Rate Data":T3)  [unwired: 6 in]
    n322 = local read "Exit Button"() -> (w637:bool)
  }
  n323 = Release Queue(queue=w48, error in (no error)=w8) -> (error out=w28:errorcluster)  [unwired: 1 in, 2 out]
  n324 = Flush Stream(8:w17, 11:w12) -> (0:w56:errorcluster, 3:w55:refnum<k21>)  [unwired: 2 in, 1 out]
  n325 = Release Queue(queue=w36, error in (no error)=w15) -> (error out=w47:errorcluster)  [unwired: 1 in, 2 out]
  n326 = Destroy Stream Endpoint(8:w56, 11:w55) -> (0:w53:errorcluster)
  n327 = Concatenate Strings(w41, "_index" ("string")) -> (w42:string)
  n328 = TDMS Flush(4:w7, 7:w51) -> (0:w49:errorcluster, 3:w50:refnum<k34>)
  n329 = String To Path(string=w42) -> (path=w40:path)
  n330 = TDMS Close(8:w49, 11:w50) -> (0:w44:errorcluster)  [unwired: 1 out]
  n331 = Delete(path (use dialog)=w40, confirm (F)=FALSE, error in=w44) -> (error out=w29:errorcluster)  [unwired: 2 in, 2 out]
  n332 = Merge Errors(w10, w29, w28, w16, w47, w53, w18, w14, w20, w19) -> (w21:errorcluster)
  n333 = flat-sequence {
    tunnel: [w657] -> w24
    tunnel: [w656] -> w22
    tunnel: w21 -> [w657]
    tunnel: w1 -> [w656]
    frame #0 {
      n334 = local write "Stop Log"(TRUE ("Stop Log")) -> ()
    }
  }
  n335 = Merge Errors(w9, w24) -> (w23:errorcluster)
  n336 = call <userlib>:"Close.vi"("error in (no error)"=w23, "EventLog ref"=w22) -> ("error out"=w25:errorcluster)  [unwired: 9 in]
  n337 = call <vilib>:"Clear Errors.vi"("error in (no error)"=w25) -> ()  [unwired: 6 in, 1 out]
